vi "ChangeGraphConfig.vi"(8 "error in (no error)":errorcluster caption="entrée d'erreur (pas d'erreur)", 10 "NewGraphConfig":u32, 11 "Interface en entrée":refnum<class "Interface.lvclass"> caption="DNL_LabVIEW Object in") -> (0 "error out":errorcluster caption="sortie d'erreur", 3 "Interface en sortie":refnum<class "Interface.lvclass"> caption="DNL_LabVIEW Object out")   [LabVIEW 2019, in "Interface.lvclass"]
uses:
  Interface.lvclass
  ChgGraphConfState.ctl
  Interface.lvclass/Interface.ctl
panel:
  out "GraphDiff":i32
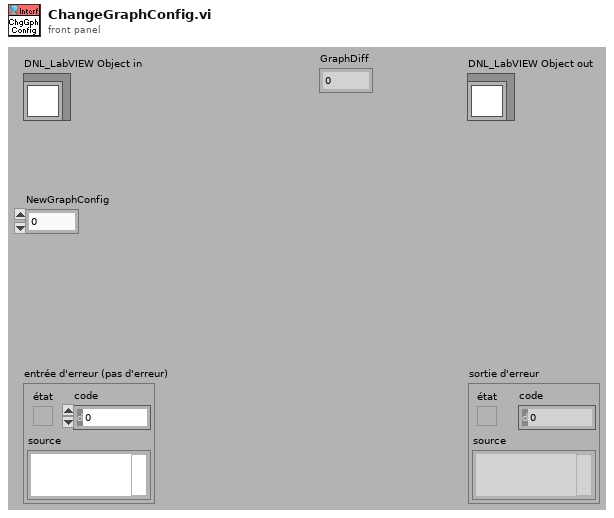
[diagram p1: front panel]
types:
  T1 = typedef "ChgGraphConfState.ctl" = enum16{"GetCurConf", "AddGraphs", "RemGraphs"}
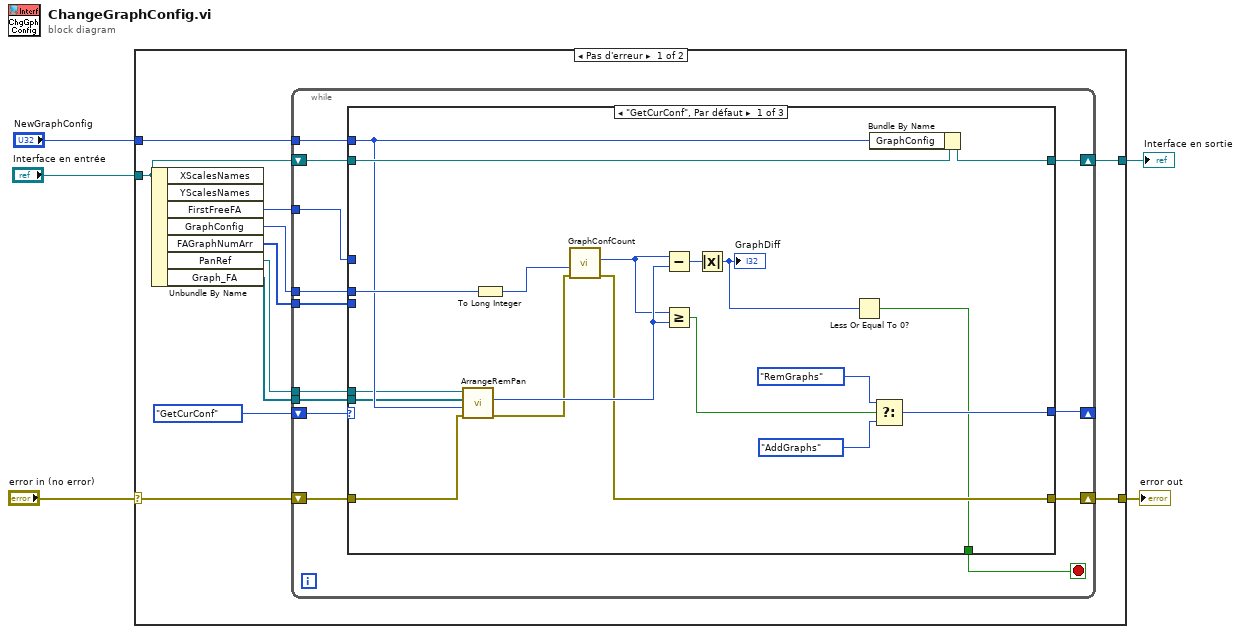
[diagram p0: block diagram]
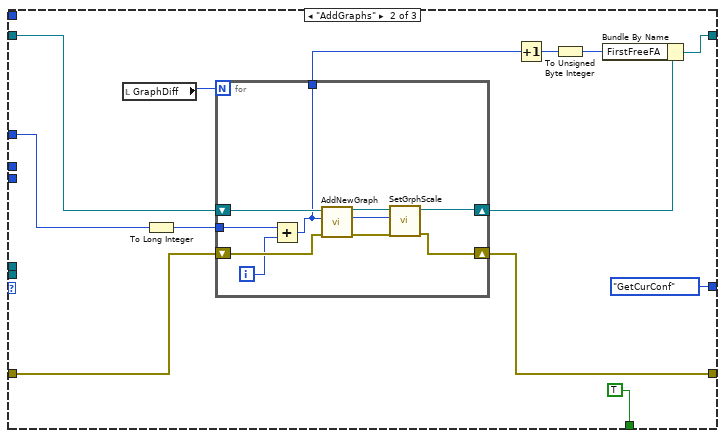
[diagram p2: hidden frame]
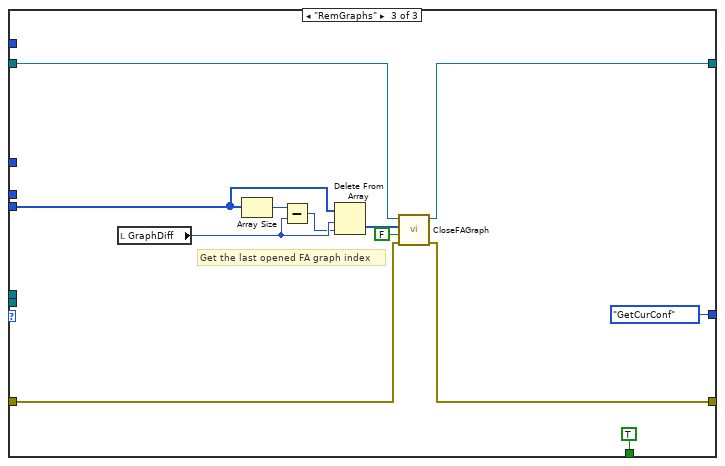
[diagram p3: hidden frame]
diagram:
  n1 = case shown="Pas d'erreur" "error in (no error)" {
    selector: "error in (no error)" -> [w11 w85]
    tunnel: [w9 w85] -> w4
    tunnel: [w8 w84] -> w2
    tunnel: "Interface en entrée" -> [w13 w84]
    tunnel: "NewGraphConfig" -> [w14 _]
    frame No Error {
      n2 = Unbundle By Name(w13) -> ("FirstFreeFA"=w12:u8, "GraphConfig"=w15:i32, "FAGraphNumArr"=w10:i32[], "PanRef"=w7:refnum<vi>, "Graph_FA"=w6:refnum<vi>[])  [unwired: 2 out]
      n3 = while {
        shift-right: [w28] -> _
        shift-left: ChgGraphConfState."GetCurConf" ("Énum") -> [w29]
        tunnel: w15 -> [w27]
        tunnel: w14 -> [w26]
        shift-right: [w21] -> w8
        shift-left: w13 -> [w25]
        tunnel: w12 -> [w24]
        shift-right: [w22] -> w9
        shift-left: w11 -> [w23]
        tunnel: w10 -> [w19]
        tunnel: w7 -> [w18]
        tunnel: w6 -> [w17]
        stop <- w20 stop-if-true
        n4 = case shown="\"GetCurConf\", Par défaut" w29 {
          tunnel: [w44 ChgGraphConfState."GetCurConf" ("Énum") ChgGraphConfState."GetCurConf" ("Énum")] -> w28
          tunnel: w27 -> [w48 _ _]
          tunnel: w26 -> [w40 _ _]
          tunnel: w25 -> [w42 w60 w82]
          tunnel: w24 -> [_ w59 _]
          tunnel: w23 -> [w39 w54 w81]
          tunnel: [w32 w53 w80] -> w22
          tunnel: [w41 w51 w77] -> w21
          tunnel: [w30 TRUE TRUE] -> w20
          tunnel: w19 -> [_ _ w83]
          tunnel: w18 -> [w37 _ _]
          tunnel: w17 -> [w36 _ _]
          frame "GetCurConf", Default {
            n5 = call "ArrangeRemPan.vi"("error in (no error)"=w39, "Configuration"=w40, "FARefArr"=w36, "PanRef"=w37) -> ("error out"=w33:errorcluster, "GraphCount"=w38:i32)  [unwired: 5 in, 1 out]
            n6 = To Long Integer(number=w48) -> (32bit integer=w35:i32)
            n7 = call "GraphConfCount.vi"("error in (no error)"=w33, "Configuration"=w35) -> ("error out"=w32:errorcluster, "GraphCount"=w34:i32)  [unwired: 8 in]
            n8 = Subtract(x=w34, y=w38) -> (x-y=w43:i32)
            n9 = Greater Or Equal?(x=w34, y=w38) -> (x >= y?=w47:bool)
            n10 = Absolute Value(x=w43) -> (abs(x)=w31:i32)
            "GraphDiff" <- w31
            n11 = Less Or Equal To 0?(x=w31) -> (x <= 0?=w30:bool)
            n12 = Bundle By Name(cluster=w42, "GraphConfig"=w40) -> (w41:refnum<class "Interface.lvclass">)
            n13 = Select(t=ChgGraphConfState."RemGraphs" ("Énum"), s=w47, f=ChgGraphConfState."AddGraphs" ("Énum")) -> (s? t:f=w44:T1)
          }
          frame "AddGraphs" {
            n14 = local read "GraphDiff"() -> (w61:i32)
            n15 = To Long Integer(number=w59) -> (32bit integer=w56:i32)
            n16 = for {
              N: w61 -> [_]
              shift-right: [w63] -> w53
              shift-left: w54 -> [w71]
              shift-right: [w62] -> w52
              shift-left: w60 -> [w70]
              tunnel: w56 -> [w68]
              tunnel: [w69] -> w58
              i -> [w67]
              n17 = Add(x=w68, y=w67) -> (x+y=w69:i32)
              n18 = call "AddNewGraph.vi"("error in (no error)"=w71, "FAIndex"=w69, "Interface en entrée"=w70) -> ("error out"=w64:errorcluster, "NewGraphInd"=w66:i32, "Interface en sortie"=w65:refnum<class "Interface.lvclass">)  [unwired: 6 in]
              n19 = call "SetGrphScale.vi"("error in (no error)"=w64, "GraphIndex"=w66, "Interface en entrée"=w65) -> ("error out"=w63:errorcluster, "Interface en sortie"=w62:refnum<class "Interface.lvclass">)  [unwired: 7 in]
            }
            n20 = Increment(x=w58) -> (x+1=w57:i32)
            n21 = To Unsigned Byte Integer(number=w57) -> (unsigned 8bit integer=w55:u8)
            n22 = Bundle By Name(cluster=w52, "FirstFreeFA"=w55) -> (w51:refnum<class "Interface.lvclass">)
          }
          frame "RemGraphs" {
            # "Get the last opened FA graph index"
            n23 = local read "GraphDiff"() -> (w76:i32)
            n24 = Array Size(array=w83) -> (size(s)=w75:i32)
            n25 = Subtract(x=w75, y=w76) -> (x-y=w73:i32)
            n26 = Delete From Array(array=w83, length=w76, index=w73) -> (deleted portion=w74:i32[])  [unwired: 1 out]
            n27 = call "CloseFAGraph.vi"("error in (no error)"=w81, "UpdtGphConf"=FALSE, "GraphIndexArr"=w74, "Interface en entrée"=w82) -> ("error out"=w80:errorcluster, "Interface en sortie"=w77:refnum<class "Interface.lvclass">)  [unwired: 6 in]
          }
        }
      }
    }
    frame Error {
    }
  }
  "error out" <- w4
  "Interface en sortie" <- w2
